vi "CalculateFromWAV.vi"(6 "Method":enum16{"Sqrt(H1H2)", "H1", "H2"}(ring), 8 "View":u16(ring) items=["Raw", "Volts", "Units (Pa, N, etc)"], 9 "Settings":T2={"Name of test"="", "Date"=timestamp(0 s since 1904-01-01), "Location"="", "Template"="", "Soundcard"="", "resolution"=32, "Sampling rate"=48000, "Ch1 Gain "=25.0, "Ch2 Gain"=10.0, "Sample time (s)"=0.3, "Pre-trigger (s)"=0.01, "Hammer Threshold"=10.0, "Positions"=12, "Taps/Position"=5, "Set Names"="", "Freq resolution"=10.0, "Hammer cutoff"=0.0, "Mic cutoff"=0.0, "Double bounce "=0.0, "Hammer Cal"=10.0, "dB Offset"=0.0, "Accel Cal"=10.0, "Vibrometer Cal"=0.0, "Mic Cal"=0.0, "Output"=2, "Voltage Cal"=1.0, "Vibrometer Port"="ASRL27::INSTR", "Range"=4, "High Pass"=2, "Bandwidth"=4, "X Range"=[], "Y Range"=[], "dB Spread"=0.0, "Trigger"=0, "Ch_1"=25, "Ch_2"=25, "flip?"=FALSE, "60Hz"=FALSE, "Time offset"=0.0, "Piezo Cal"=1.0, "Default Notes"=""} {"Ch_2" min=1 step=1; "Ch_1" min=1 max=100 step=1; "Trigger" items=["Hammer (force)", "Self-tap", "Spacebar"]; "Bandwidth" items=["1 kHz"=1, "5 kHz"=5, "10 kHz"=10, "25 kHz"=25, "50 kHz"=50, "100 kHz"=100]; "High Pass" items=["Off", "13 Hz", "104 Hz"]; "Range" items=["10 mm/s"=1, "20 mm/s"=2, "50 mm/s"=5, "100 mm/s"=10, "200 mm/s"=20, "500 mm/s"=50, "1 m/s"=100, "2 m/s"=200]; "Output" items=["Accelerometer", "Speed (from acceleration)", "Microphone", "Vibrometer", "Piezo"]; "Voltage Cal" format="%#_13g"; "Ch2 Gain" format="%#_13g"; "Ch1 Gain" format="%#_13g"; "Double bounce" min=0.0; "Mic cutoff" min=0.0 format="%#_4g"; "Hammer cutoff" min=0.0 format="%#_4g"; "Freq resolution" min=0.0; "Pre-trigger (s)" format="%#_13g"; "Date" format="%<%H:%M\n%d/%m/%y>T"; "resolution" items=["16 bit"=16, "24 bit"=24, "32 bit"=32]; "Sampling rate" items=["22050 samp/s"=22050, "44100 samp/s"=44100, "48000 samp/s"=48000]}, 10 "path":path) -> (0 "Plots":T1, 1 "trf file":path, 2 "Alert":string, 3 "Last Data Set":waveform(dbl)[](array[waveform]), 4 "Old FRFs":cluster{dbl, "dt":dbl, "Y":dbl[]}[](graph))   [LabVIEW 2022 SP3]
uses:
  PreferencesControl.ctl
panel:
  out "Array":path[](array[path])
  # "Hz"
  # "dB"
  # "dB"
  # "sec"
  # "sec"
  # "mV/Pa"
  # "mV/m/s2"
  # "mV/mm/s"
  # "V/N"
  # "sec"
  # "sec"
  # "mV/N"
  # "a.u."
  # "a.u."
  # "sec"
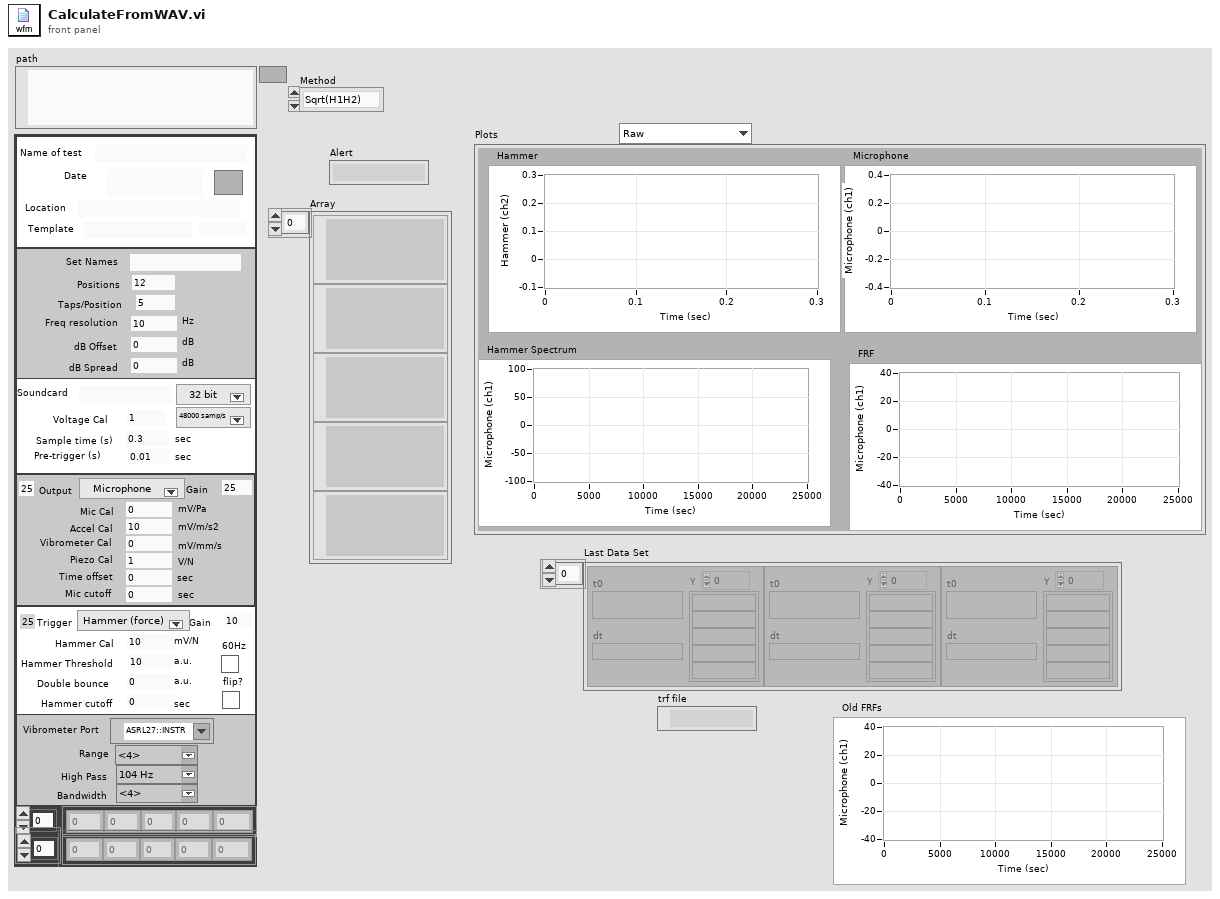
[diagram p1: front panel]
types:
  T1 = cluster{"Hammer":cluster{dbl, "dt":dbl, "Y":dbl[]}[], "Microphone":cluster{dbl, "dt":dbl, "Y":dbl[]}[], "Hammer Spectrum":cluster{dbl, "dt":dbl, "Y":dbl[]}[], "FRF":cluster{dbl, "dt":dbl, "Y":dbl[]}[]}
  T2 = typedef "PreferencesControl.ctl" = cluster{"Name of test":string, "Date":timestamp, "Location":string, "Template":string, "Soundcard":string, "resolution":u16, "Sampling rate":u16, "Ch1 Gain ":dbl, "Ch2 Gain":dbl, "Sample time (s)":dbl, "Pre-trigger (s)":dbl, "Hammer Threshold":dbl, "Positions":i16, "Taps/Position":i16, "Set Names":string, "Freq resolution":dbl, "Hammer cutoff":dbl, "Mic cutoff":dbl, "Double bounce ":dbl, "Hammer Cal":dbl, "dB Offset":dbl, "Accel Cal":dbl, "Vibrometer Cal":dbl, "Mic Cal":dbl, "Output":u16, "Voltage Cal":dbl, "Vibrometer Port":refnum<visa-resource-name>, "Range":u16, "High Pass":u16, "Bandwidth":u16, "X Range":cluster{"Minimum":dbl, "Maximum":dbl, "Increment":dbl, "Minor Increment":dbl, "Start":dbl}[], "Y Range":cluster{"Minimum":dbl, "Maximum":dbl, "Increment":dbl, "Minor Increment":dbl, "Start":dbl}[], "dB Spread":dbl, "Trigger":u16, "Ch_1":u8, "Ch_2":u8, "flip?":bool, "60Hz":bool, "Time offset":dbl, "Piezo Cal":dbl, "Default Notes":string}
  T3 = cluster{"Test":string, "Set":string, "Position":string, "Tap":string}
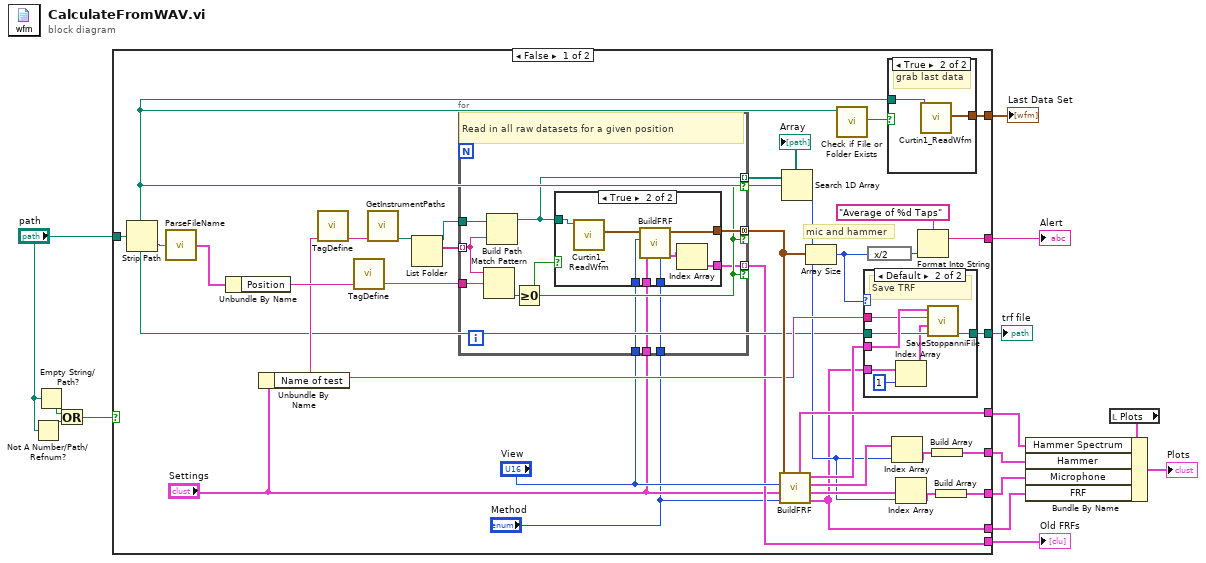
[diagram p0: block diagram]
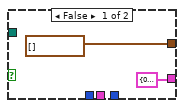
[diagram p4: hidden frame]
diagram:
  n1 = Not A Number/Path/Refnum?(number/path/refnum="path") -> (NaN/Path/Refnum?=w13:bool)
  n2 = Empty String/Path?(string/path="path") -> (empty?=w12:bool)
  n3 = Or(x=w12, y=w13) -> (x .or. y?=w11:bool)
  n4 = case shown="False" w11 {
    tunnel: [w47 _] -> w14
    tunnel: [w46 _] -> w10
    tunnel: [w20 _] -> w7
    tunnel: [w32 _] -> w9
    tunnel: [w29 _] -> w8
    tunnel: "path" -> [w22 _]
    tunnel: [w26 _] -> w3
    tunnel: [w18 _] -> w2
    tunnel: [w15 _] -> w1
    frame False {
      # "mic and hammer"
      n5 = Strip Path(path=w22) -> (name=w44:string)  [unwired: 1 out]
      n6 = call "ParseFileName.vi"("String in"=w44) -> ("Name"=w45:T3)  [unwired: 2 out]
      n7 = Unbundle By Name(w45) -> ("Position"=w37:string)
      n8 = Unbundle By Name("Settings") -> ("Name of test"=w27:string)
      n9 = call "TagDefine.vi"("LUT in"=w27) -> ("String Out"=w38:string)  [unwired: 9 in, 1 out]
      n10 = call "TagDefine.vi"("LUT in"=w37) -> ("String Out"=w39:string)  [unwired: 9 in, 1 out]
      n11 = call "GetInstrumentPaths.vi"("Instrument"=w38) -> ("Path To Raw Folder"=w42:path)  [unwired: 6 in, 4 out]
      n12 = List Folder(path=w42) -> (path out=w40:path, filenames=w41:string[])  [unwired: 3 in, 2 out]
      n13 = for {
        tunnel: w41 -> [w64] mode=indexing
        tunnel: w39 -> [w67]
        tunnel: w40 -> [w65]
        tunnel: [w62] -> w43 mode=concatenating if=w61
        tunnel: [w63] -> w25 mode=indexing if=w61
        tunnel: "View" -> [w58]
        tunnel: [w57] -> w18 mode=indexing if=w61
        tunnel: "Settings" -> [w59]
        tunnel: "Method" -> [w60]
        # "Read in all raw datasets for a given position"
        n14 = Match Pattern(string=w64, regular expression=w67) -> (offset past match=w66:i32)  [unwired: 1 in, 3 out]
        n15 = Build Path(base path=w65, name or relative path=w64) -> (appended path=w63:path)
        n16 = Greater Or Equal To 0?(x=w66) -> (x >= 0?=w61:bool)
        n17 = case shown="True" w61 {
          tunnel: w63 -> [_ w76]
          tunnel: [waveform(dbl)[] [] ("all waveforms in record") w75] -> w62
          tunnel: w60 -> [_ w73]
          tunnel: w59 -> [_ w72]
          tunnel: w58 -> [_ w71]
          tunnel: [cluster{dbl, "df":dbl, dbl[]} {0.0, "df"=0.0, []} w70] -> w57
          frame False {
          }
          frame True {
            n18 = call "Curtin1_ReadWfm.vi"("appended path"=w76) -> ("all waveforms in record"=w75:waveform(dbl)[])  [unwired: 9 in, 1 out]
            n19 = call "BuildFRF.vi"("Method"=w73, "Settings"=w72, "View"=w71, "Data In"=w75) -> ("Average FRF"=w74:cluster{dbl, "df":dbl, dbl[]}[])  [unwired: 2 in, 5 out]
            n20 = Index Array(array=w74) -> (element=w70:cluster{dbl, "df":dbl, dbl[]})  [unwired: 1 in]
          }
        }
      }
      "Array" <- w25
      n21 = call "BuildFRF.vi"("Method"="Method", "Settings"="Settings", "View"="View", "Data In"=w43) -> ("Average FRF"=w20:cluster{dbl, "df":dbl, dbl[]}[], "Microphone"=w30:cluster{dbl, "dt":dbl, "Y":dbl[]}[], "Hammer"=w33:cluster{dbl, "dt":dbl, "Y":dbl[]}[], "Complex FRF"=w28:cluster{"t0":dbl, "dt":dbl, "Y":cdb[]}, "Hammer Spectra"=w46:cluster{dbl, "df":dbl, "FFT {X}":dbl[]}[])  [unwired: 2 in, 1 out]
      n22 = Search 1D Array(1D array=w25, element=w22) -> (index of element=w24:i32)  [unwired: 1 in]
      n23 = Array Size(array=w43) -> (size(s)=w23:i32)
      n24 = call <vilib>:"Check if File or Folder Exists.vi"("path"=w22) -> ("file or folder exists?"=w21:bool)  [unwired: 8 in, 2 out]
      n25 = case shown="Default" w23 {
        tunnel: w28 -> [_ w56]
        tunnel: w27 -> [_ w55]
        tunnel: w22 -> [_ w54]
        tunnel: w20 -> [_ w53]
        tunnel: [_ w50] -> w15
        frame 0 {
        }
        frame Default {
          # "Save TRF"
          n26 = Index Array(array=w53, index=1) -> (element=w52:cluster{dbl, "df":dbl, dbl[]})
          n27 = call "SaveStoppanniFile.vi"("Last Path"=w54, "Coherence in"=w52, "Inst:Test Name"=w55, "Complex FRF"=w56) -> ("trf file"=w50:path)  [unwired: 7 in]
        }
      }
      n28 = expression code="x/2"(w23) -> (w35:i32)
      n29 = case shown="True" w21 {
        tunnel: [_ w48] -> w26
        tunnel: w22 -> [_ w49]
        frame False {
        }
        frame True {
          # "grab last data"
          n30 = call "Curtin1_ReadWfm.vi"("appended path"=w49) -> ("all waveforms in record"=w48:waveform(dbl)[])  [unwired: 9 in, 1 out]
        }
      }
      n31 = Index Array(array=w33, index=w24) -> (element=w34:cluster{dbl, "dt":dbl, "Y":dbl[]})
      n32 = Index Array(array=w30, index=w24) -> (element=w31:cluster{dbl, "dt":dbl, "Y":dbl[]})
      n33 = Format Into String(format string="Average of %d Taps", w35) -> (resulting string=w47:string)  [unwired: 2 in, 1 out]
      n34 = Build Array(w34) -> (w32:cluster{dbl, "dt":dbl, "Y":dbl[]}[])
      n35 = Build Array(w31) -> (w29:cluster{dbl, "dt":dbl, "Y":dbl[]}[])
    }
    frame True {
    }
  }
  "Alert" <- w14
  "Last Data Set" <- w3
  "Old FRFs" <- w2
  "trf file" <- w1
  n36 = local read "Plots"() -> (w6:T1)
  n37 = Bundle By Name(cluster=w6, "Hammer Spectrum"=w10, "Hammer"=w9, "Microphone"=w8, "FRF"=w7) -> (→"Plots":T1)
